vi "StartVIserver.vi"(8 "error in (no error)":errorcluster, 11 "Application Ref":refnum<vi>) -> (0 "error out":errorcluster, 2 "Port":u32, 3 "Application Ref Out":refnum<vi>)   [LabVIEW 2012, in "DataProcessingToolkit.lvlib"]
uses:
  DataProcessingToolkit.lvlib
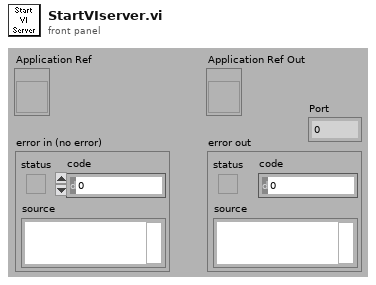
[diagram p1: front panel]
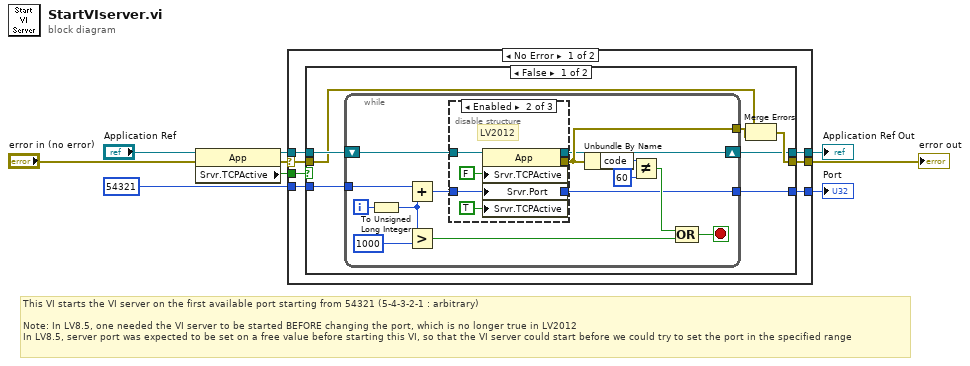
[diagram p0: block diagram]
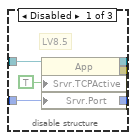
[diagram p2: hidden frame]
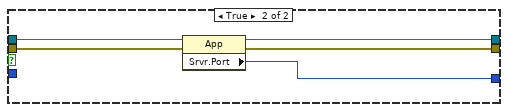
[diagram p4: hidden frame]
diagram:
  # "This VI starts the VI server on the first available port starting from 54321 (5-4-3-2-1 : arbitrary)\n\nNote: In LV8.5, one needed the VI server to be started BEFORE changing the port, which is no longer true in LV2012\nIn LV8.5, server port was expected to be set on a free value before starting this VI, so that the VI server could start before we could try to set the port in the specified range"
  n1 = property class="App"(reference="Application Ref", error in="error in (no error)") -> (reference out=w8:refnum<vi>, error out=w9:errorcluster, "Srvr.TCPActive"=w1:bool)
  n2 = case shown="No Error" w9 {
    selector: w9 -> [w14 w56]
    tunnel: u32 54321 ("Srvr.Port") -> [w16 w54]
    tunnel: w8 -> [w15 w55]
    tunnel: [w13 w56] -> w7
    tunnel: [w12 w55] -> w6
    tunnel: [w11 w54] -> w5
    tunnel: w1 -> [w10 _]
    frame No Error {
      n3 = case shown="False" w10 {
        tunnel: w16 -> [w23 _]
        tunnel: w15 -> [w22 w53]
        tunnel: w14 -> [w20 w52]
        tunnel: [w19 w50] -> w13
        tunnel: [w18 w51] -> w12
        tunnel: [w17 w49] -> w11
        frame False {
          n4 = while {
            tunnel: w23 -> [w26]
            shift-right: [w27] -> w18
            shift-left: w22 -> [w28]
            tunnel: [w31] -> w21
            tunnel: [w29] -> w17
            i -> [w30]
            stop <- w33 stop-if-true
            n5 = To Unsigned Long Integer(number=w30) -> (unsigned 32bit integer=w25:u32)
            n6 = Add(x=w26, y=w25) -> (x+y=w24:u32)
            n7 = Greater?(x=w25, y=u32 1000) -> (0:w36:bool)
            n8 = disable-structure shown="Enabled" {
              disable-tunnel: [w42 w48 _] -> w31
              disable-tunnel: [w38 w43 _] -> w29
              disable-tunnel: w28 -> [w40 w46 _]
              disable-tunnel: [w39 w45 _] -> w27
              disable-tunnel: w24 -> [w38 w43 _]
              frame Disabled {
                # "LV8.5"
                n9 = property class="App"(reference=w40, "Srvr.TCPActive"=TRUE ("Server:TCP Listener Active"), "Srvr.Port"=w38) -> (reference out=w39:refnum<vi>, error out=w42:errorcluster)  [unwired: 1 in]
              }
              frame Enabled {
                # "LV2012"
                n10 = property class="App"(reference=w46, "Srvr.TCPActive"=FALSE ("Server:TCP Listener Active"), "Srvr.Port"=w43, "Srvr.TCPActive"=TRUE ("Server:TCP Listener Active")) -> (reference out=w45:refnum<vi>, error out=w48:errorcluster)  [unwired: 1 in]
              }
              frame Disabled {
              }
            }
            n11 = Unbundle By Name(w31) -> ("code"=w35:i32)
            n12 = Not Equal?(x=w35, y=60) -> (x != y?=w32:bool)
            n13 = Compound Arithmetic op=OR(w32, w36) -> (w33:bool)
          }
          n14 = Merge Errors(w20, w21) -> (w19:errorcluster)
        }
        frame True {
          n15 = property class="App"(reference=w53, error in=w52) -> (reference out=w51:refnum<vi>, error out=w50:errorcluster, "Srvr.Port"=w49:u32)
        }
      }
    }
    frame Error {
    }
  }
  "error out" <- w7
  "Application Ref Out" <- w6
  "Port" <- w5
